vi "Test Quaternion Conversion.vi"(11 "Test Case In":refnum<class "03_AR.lvclass">) -> (0 "error out":errorcluster, 3 "Test Case Out":refnum<class "03_AR.lvclass">)   [LabVIEW 2020, in "test.lvlib" / "03_AR.lvclass"]
uses:
  03_AR.lvclass
  C:/Program Files (x86)/National Instruments/LabVIEW 2026/vi.lib/Astemes/LUnit/Test Case.lvclass
  <vilib>/Analysis/Matrix/Datatypes/RealMatrix.ctl
  ar/Quaternion.ctl
  <vilib>/Astemes/LUnit/Test Case.lvclass/Test Case.ctl
  4993e8ee-a06a-463a-9684-69129f64d5ce.vi
  <vilib>/Astemes/LUnit/Core/LUnit Test Case/Private/Append Pass Result.vi
  <vilib>/Astemes/LUnit/Core/LUnit Test Case/Private/Append Fail Result.vi
  4993e8ee-a06a-463a-9684-69129f64d5ce.vi/9c5d11cd-9439-4240-a1ee-d9baace9c924.vi
  <vilib>/Astemes/LUnit/Core/LUnit Test Case/Private/Run In UI.vi
  <vilib>/Utility/error.llb/Clear Errors.vi
  <vilib>/Utility/error.llb/Error Cluster From Error Code.vi
  <vilib>/Analysis/Matrix/Numeric/Conversions/Array To Matrix.vi
  <vilib>/Analysis/Matrix/Numeric/Conversions/Array To Matrix - RA2.vi
  <vilib>/Analysis/Matrix/Numeric/Subtract/Subtract - RM,RM.vi
  <vilib>/Analysis/Matrix/Numeric/Absolute Value/Absolute Value - RM.vi
  ar/ar.lvlib
  <vilib>/Analysis/Matrix/NI_Matrix.lvlib
  <vilib>/Astemes/LUnit/Test Case.lvclass
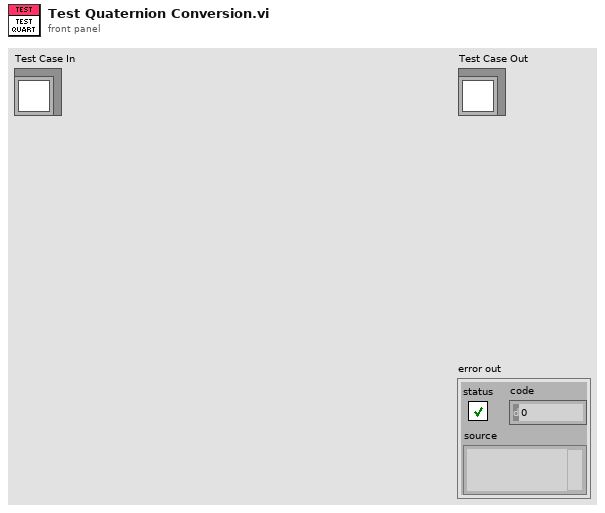
[diagram p1: front panel]
types:
  T1 = typedef "ar.lvlib/Quaternion.ctl" = cluster{"w":dbl, "x":dbl, "y":dbl, "z":dbl}
  T2 = typedef "NI_Matrix.lvlib/RealMatrix.ctl" = dbl[][]
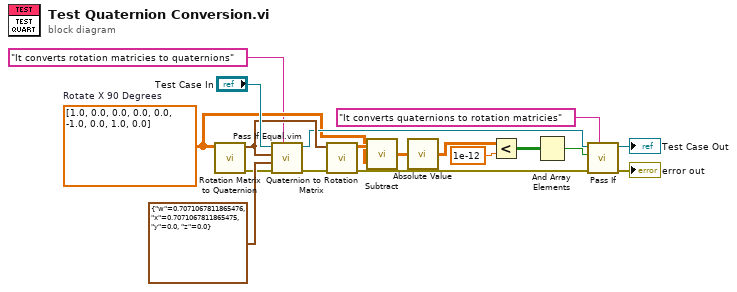
[diagram p0: block diagram]
diagram:
  w8 = T2 [[1.0, 0.0, 0.0], [0.0, 0.0, -1.0], [0.0, 1.0, 0.0]]  # Rotate X 90 Degrees
  n1 = call "Rotation Matrix to Quaternion.vi"("Rotation Matrix"=w8) -> ("error out"=w10:errorcluster, "Quaternion"=w17:T1)  [unwired: 9 in]
  n2 = call "Pass If Equal.vim"("Description"="It converts rotation matricies to quaternions", "error in (no error)"=w10, "Actual"=T1 {"w"=0.7071067811865476, "x"=0.7071067811865475, "y"=0.0, "z"=0.0} ("Quaternion"), "Expected"=w17, "LUnit Test Case In"="Test Case In") -> ("error out"=w12:errorcluster, "LUnit Test Case Out"=w14:refnum<class "03_AR.lvclass">)  [unwired: 5 in]
  n3 = call "Quaternion to Rotation Matrix.vi"("error in (no error)"=w12, "Quaternion"=w17) -> ("error out"=w11:errorcluster, "Rotation Matrix"=w9:T2)  [unwired: 8 in]
  n4 = call-poly <vilib>:"Subtract.vi"("Real Matrix B"=w8, "Real Matrix A"=w9) -> ("A - B"=w7:T2)
  n5 = call-poly <vilib>:"Absolute Value.vi"("Real Matrix A"=w7) -> ("|A|"=w6:T2)
  n6 = Less?(x=w6, y=1e-12) -> (x < y?=w4:bool[][])
  n7 = And Array Elements(Boolean array=w4) -> (logical AND=w3:bool)
  n8 = call <vilib>:"Pass If.vi"("Description"="It converts quaternions to rotation matricies", "error in (no error)"=w11, "Pass?"=w3, "LUnit Test Case In"=w14) -> ("error out"=→"error out":errorcluster, "LUnit Test Case Out"=→"Test Case Out":refnum<class "03_AR.lvclass">)  [unwired: 6 in]
